vi "Start Move.vi"(8 "error in (no error)":errorcluster, 10 "Coords":T1, 11 "SwipeScrollListbox in":refnum<class "SwipeScrollListbox.lvclass">) -> (0 "error out":errorcluster, 2 "Button Down":bool, 3 "SwipeScrollListbox out":refnum<class "SwipeScrollListbox.lvclass">)   [LabVIEW 2020, in "SwipeScrollListbox.lvclass"]
uses:
  SwipeScrollListbox.lvclass
  C:/Program Files/National Instruments/LabVIEW 2020/vi.lib/QSI/QControls/QControl Classes/ListBox/ListBox.lvclass
  <vilib>/Utility/miscctls.llb/LVPoint32TypeDef.ctl
  SwipeScrollListbox.lvclass/SwipeScrollListbox.ctl
  <vilib>/Utility/inputDevices.llb/mouseAcquire.vi
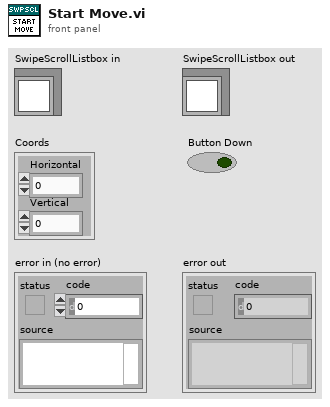
[diagram p1: front panel]
types:
  T1 = typedef "LVPoint32TypeDef.ctl" = cluster{"Horizontal":i32, "Vertical":i32}
  T2 = cluster{"Horizontal":i32, "Vertical":i32, "Scrolling":i32}
  T3 = cluster{"button 1":bool, "button 2":bool, "button 3":bool, "button 4":bool}
  T4 = typedef "SwipeScrollListbox.lvclass/State Data.ctl" = cluster{"Timeout":i32, "Time":timestamp, "Y":i32, "Slow Distance":i32, "Rate":dbl, "Row Selected":i32}
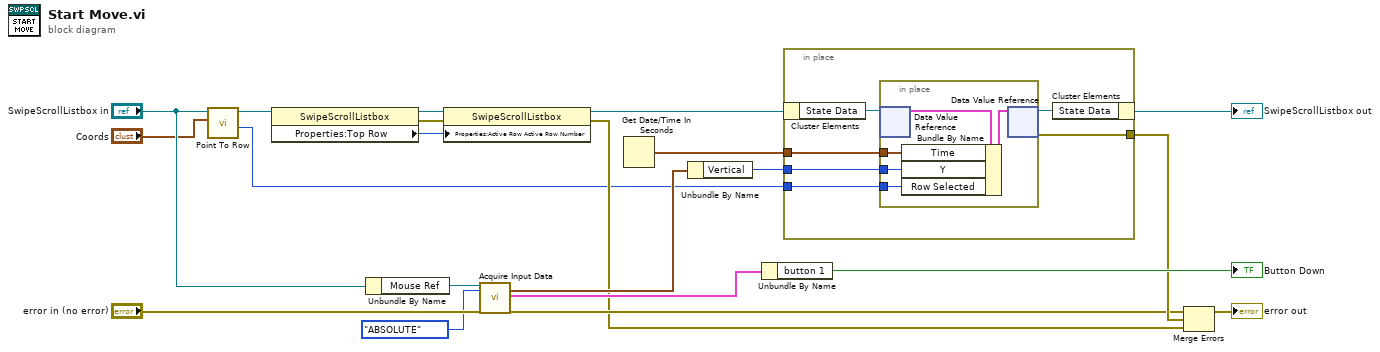
[diagram p0: block diagram]
diagram:
  n1 = call-dynamic "Point To Row.vi"("Point"="Coords", "ListBox in"="SwipeScrollListbox in") -> ("Row"=w1:i32, "ListBox out"=w3:refnum<class "SwipeScrollListbox.lvclass">)  [unwired: 5 in, 3 out]
  n2 = property class="SwipeScrollListbox"(reference=w3) -> (reference out=w8:refnum<class "SwipeScrollListbox.lvclass">, error out=w7:errorcluster, "Properties:Top Row"=w6:i32)  [unwired: 1 in]
  n3 = Unbundle By Name("SwipeScrollListbox in") -> ("Mouse Ref"=w16:refnum<k1>)
  n4 = property class="SwipeScrollListbox"(reference=w8, error in=w7, "Properties:Active Row Active Row Number"=w6) -> (reference out=w9:refnum<class "SwipeScrollListbox.lvclass">, error out=w10:errorcluster)
  n5 = call-poly <vilib>:"Acquire Input Data.vi"("device ID"=w16, "key mode"=enum16{"RELATIVE", "ABSOLUTE"}."ABSOLUTE", "error in (no error)"="error in (no error)") -> ("axis info"=w12:T2, "button info"=w13:T3, "error out"=w14:errorcluster)  [unwired: 13 in, 1 out]
  n6 = Get Date/Time In Seconds() -> (seconds since 1Jan1904=w19:timestamp)
  n7 = Unbundle By Name(w12) -> ("Vertical"=w11:i32)
  n8 = Unbundle By Name(w13) -> ("button 1"=→"Button Down":bool)
  n9 = in-place {
    in-place-border: w19 -> [w25]
    in-place-border: w11 -> [w24]
    in-place-border: [w23] -> w17
    in-place-border: w1 -> [w22]
    n10 = in-place-cluster #1(w9) -> ("State Data"=w27:refnum<data-value>)
    n11 = in-place {
      in-place-border: w25 -> [w30]
      in-place-border: w24 -> [w29]
      in-place-border: w22 -> [w28]
      n12 = in-place-dvr #2(w27) -> (w32:T4)  [unwired: 1 out]
      n13 = Bundle By Name(cluster=w32, "Time"=w30, "Y"=w29, "Row Selected"=w28) -> (w31:T4)
      n14 = in-place-dvr #2(w31) -> (w26:refnum<data-value>, w23:errorcluster)
    }
    n15 = in-place-cluster #1("State Data"=w26) -> (→"SwipeScrollListbox out":refnum<class "SwipeScrollListbox.lvclass">)
  }
  n16 = Merge Errors(w14, w17, w10) -> (→"error out":errorcluster)
